vi "Add Channel.vi"(4 "SignalID":i32, 6 "Faultable":bool, 7 "GUID (Default Channel)":string="03D3BB99-1485-13A6-561D1F898F032919", 8 "error in":errorcluster, 9 "Channel Type":T2, 10 "Channel Name":string, 11 "Parent Ref in":T1 format="%.0x") -> (0 "error out":errorcluster, 2 "Channel Ref":T1 format="%.0x", 3 "Parent Ref out":T1 format="%.0x")   [LabVIEW 2026, in "NIVS Runtime Configuration File Scripting API.lvlib"]
uses:
  NIVS Runtime Configuration File Scripting API.lvlib
  <vilib>/NI VeriStand/Custom Device API/Custom Device Item Ref.ctl
  <vilib>/NI VeriStand/Custom Device API/Custom Device Channel Type.ctl
  <vilib>/NI VeriStand/Custom Device API/Custom Device Channel.ctl
  <vilib>/NI VeriStand/Custom Device API/Custom Device API.lvlib
  <vilib>/NI VeriStand/Custom Device Offline API/Custom Device Offline API.lvlib
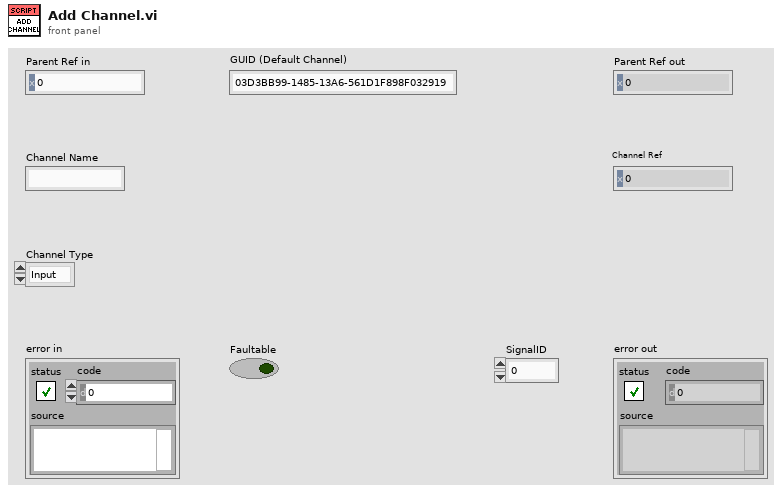
[diagram p1: front panel]
types:
  T1 = typedef "Custom Device API.lvlib/Custom Device Item Ref.ctl" = u64
  T2 = typedef "Custom Device API.lvlib/Custom Device Channel Type.ctl" = enum16{"Input", "Output"}
  T3 = typedef "Custom Device API.lvlib/Custom Device Channel.ctl" = cluster{"Type":T2, "Units":string, "Default Value":dbl, "Faultable":bool, "Scalable":bool}
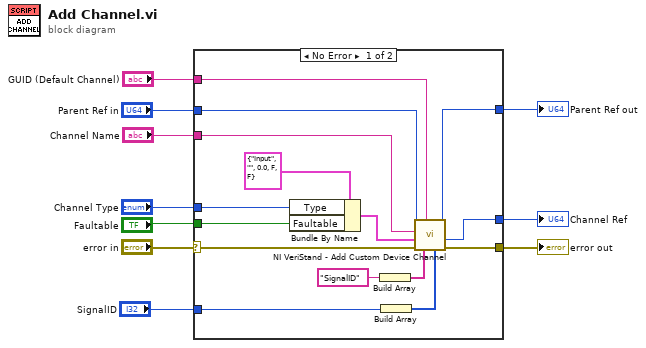
[diagram p0: block diagram]
diagram:
  n1 = case shown="No Error" "error in" {
    selector: "error in" -> [w24 w27]
    tunnel: "Parent Ref in" -> [w23 w26]
    tunnel: "Channel Name" -> [w22 _]
    tunnel: [w21 w26] -> w6
    tunnel: [w25 w27] -> w10
    tunnel: [w20 _] -> w5
    tunnel: "Channel Type" -> [w18 _]
    tunnel: "Faultable" -> [w17 _]
    tunnel: "SignalID" -> [w14 _]
    tunnel: "GUID (Default Channel)" -> [w12 _]
    frame No Error {
      n2 = Bundle By Name(cluster=T3 {"Type"=enum."Input", "Units"="", "Default Value"=0.0, "Faultable"=FALSE, "Scalable"=FALSE} ("Channel"), "Type"=w18, "Faultable"=w17) -> (w11:T3)
      n3 = Build Array("SignalID") -> (w16:string[])
      n4 = Build Array(w14) -> (w13:i32[])
      n5 = call <vilib>:"NI VeriStand - Add Custom Device Channel.vi"("Property Values"=w13, "Property names"=w16, "GUID (Default Channel)"=w12, "error in (no error)"=w24, "Channel"=w11, "Channel Name"=w22, "Parent Ref in"=w23) -> ("error out"=w25:errorcluster, "Channel Ref"=w20:T1, "Parent Ref out"=w21:T1)  [unwired: 1 in, 1 out]
    }
    frame Error {
    }
  }
  "Parent Ref out" <- w6
  "error out" <- w10
  "Channel Ref" <- w5
